vi "global_main.vi"() -> ()   [LabVIEW 2018]
uses:
  global.vi
panel:
  in  "정지 버튼":bool
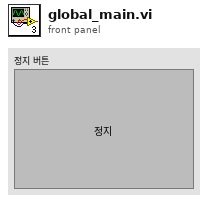
[diagram p1: front panel]
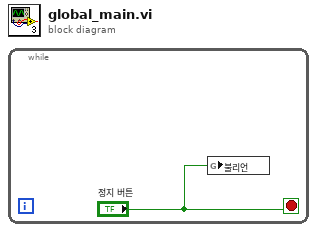
[diagram p0: block diagram]
diagram:
  n1 = while {
    stop <- "정지 버튼" stop-if-true
    n2 = global write "global.vi" "불리언"("정지 버튼") -> ()
  }
